vi "Execute.vi"(8 "error in":errorcluster, 9 "Consumer Queues in":T1, 10 "DAC Process Command in":refnum<class "Generic DAC Process Command.lvclass">, 11 "DAC Process Data in":T2) -> (0 "error out":errorcluster, 1 "Consumer Queues out":T1, 2 "Stop?":bool, 3 "DAC Process Data out":T2)   [LabVIEW 2019, in "DAC Process.lvlib" / "Generic DAC Process Command.lvclass"]
uses:
  Generic DAC Process Command.lvclass
  DAC Process Data.ctl
  Generic Test Stand/Generic Test Stand.lvclass
  TS Framework/ExeLogging/DAC Logger/DAC Logger.lvclass
  DAC State.ctl
  TS Framework/Consumer Queues.ctl
  UI Process/Generic UI Command/Generic UI Process Command.lvclass
  Trig Process/Generic Trig Command/Generic Trig Process Command.lvclass
  Generic DAC Process Command.lvclass/Generic DAC Process Command.ctl
  DAC Process.lvlib
  TS Framework/TS Framework.lvlib
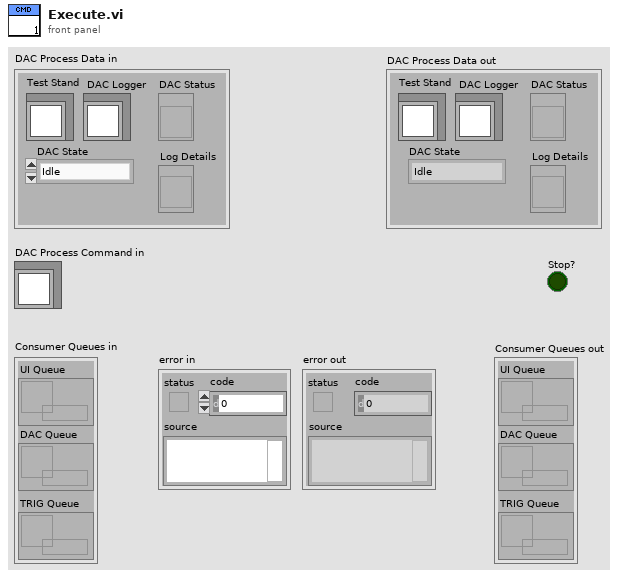
[diagram p1: front panel]
types:
  T1 = typedef "TS Framework.lvlib/Consumer Queues.ctl" = cluster{"UI Queue":refnum<queue>, "DAC Queue":refnum<queue>, "TRIG Queue":refnum<queue>}
  T2 = typedef "DAC Process.lvlib/DAC Process Data.ctl" = cluster{"Test Stand":refnum<class "Generic Test Stand.lvclass">, " DAC Logger":refnum<class "DAC Logger.lvclass">, "DAC State":T3, "DAC Status":refnum<vi>, "Log Details":refnum<vi>}
  T3 = typedef "DAC Process.lvlib/DAC State.ctl" = enum16{"Idle", "Acquiring"}
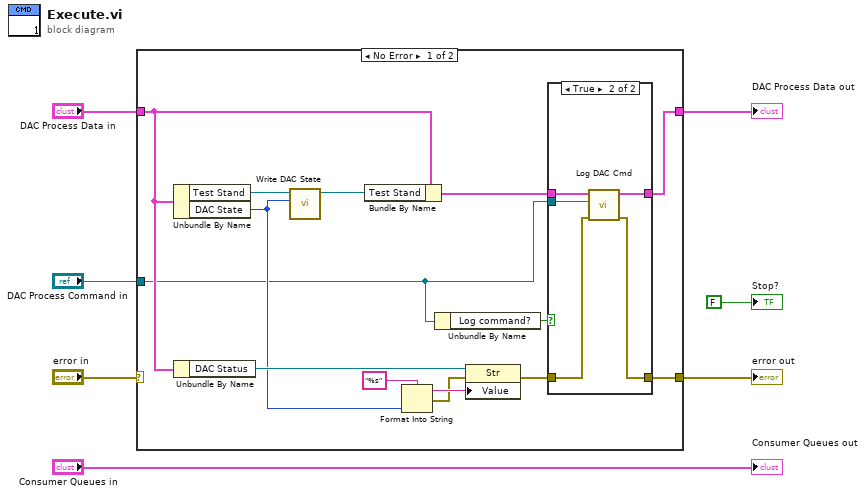
[diagram p0: block diagram]
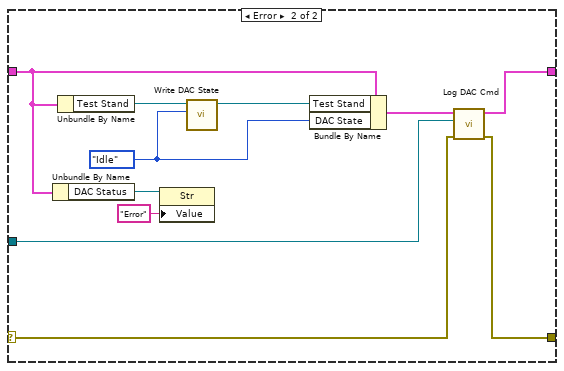
[diagram p3: hidden frame]
diagram:
  n1 = case shown="No Error" "error in" {
    selector: "error in" -> [_ w38]
    tunnel: "DAC Process Data in" -> [w13 w31]
    tunnel: "DAC Process Command in" -> [w8 w39]
    tunnel: [w20 w37] -> w3
    tunnel: [w19 w29] -> w2
    frame No Error {
      n2 = Unbundle By Name(w13) -> ("Test Stand"=w12:refnum<class "Generic Test Stand.lvclass">, "DAC State"=w11:T3)
      n3 = Unbundle By Name(w13) -> ("DAC Status"=w17:refnum<vi>)
      n4 = call "Write DAC State.vi"("DAC State"=w11, "Generic Test Stand in"=w12) -> ("Generic Test Stand out"=w9:refnum<class "Generic Test Stand.lvclass">)  [unwired: 8 in, 1 out]
      n5 = Bundle By Name(cluster=w13, "Test Stand"=w9) -> (w10:T2)
      n6 = Format Into String(format string="%s", w11) -> (resulting string=w16:string, error out=w15:errorcluster)  [unwired: 2 in]
      n7 = Unbundle By Name(w8) -> ("Log command?"=w21:bool)
      n8 = property class="Str"(reference=w17, error in=w15, "Value"=w16) -> (error out=w14:errorcluster)  [unwired: 1 out]
      n9 = case shown="True" w21 {
        tunnel: w10 -> [w22 w27]
        tunnel: w8 -> [_ w28]
        tunnel: w14 -> [w23 w26]
        tunnel: [w22 w24] -> w19
        tunnel: [w23 w25] -> w20
        frame False {
          # "Don't log this command"
        }
        frame True {
          # "Log this command"
          n10 = call "Log DAC Cmd.vi"("error in"=w26, "DAC Process Command in"=w28, "DAC Process Data in"=w27) -> ("error out"=w25:errorcluster, "DAC Process Data out"=w24:T2)  [unwired: 7 in]
        }
      }
    }
    frame Error {
      w32 = DAC_State."Idle" ("DAC State")
      # "Error - Log all commands"
      n11 = Unbundle By Name(w31) -> ("DAC Status"=w36:refnum<vi>)
      n12 = Unbundle By Name(w31) -> ("Test Stand"=w33:refnum<class "Generic Test Stand.lvclass">)
      n13 = property class="Str"(reference=w36, "Value"="Error") -> ()  [unwired: 1 in, 2 out]
      n14 = call "Write DAC State.vi"("DAC State"=w32, "Generic Test Stand in"=w33) -> ("Generic Test Stand out"=w34:refnum<class "Generic Test Stand.lvclass">)  [unwired: 8 in, 1 out]
      n15 = Bundle By Name(cluster=w31, "Test Stand"=w34, "DAC State"=w32) -> (w30:T2)
      n16 = call "Log DAC Cmd.vi"("error in"=w38, "DAC Process Command in"=w39, "DAC Process Data in"=w30) -> ("error out"=w37:errorcluster, "DAC Process Data out"=w29:T2)  [unwired: 7 in]
    }
  }
  "error out" <- w3
  "DAC Process Data out" <- w2
  "Stop?" <- FALSE
  "Consumer Queues out" <- "Consumer Queues in"
